vi "test.vi"   [LabVIEW 2015]
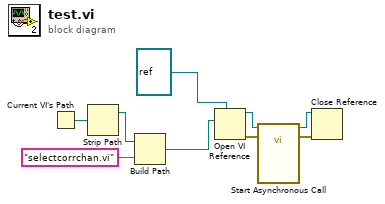
[diagram p0: block diagram]
diagram:
  n1 = Current VI's Path() -> (path=w9:path)
  n2 = Strip Path(path=w9) -> (stripped path=w5:path)  [unwired: 1 out]
  n3 = Build Path(base path=w5, name or relative path="selectcorrchan.vi") -> (appended path=w4:path)
  n4 = Open VI Reference(type specifier VI Refnum (for type only)=refnum<vi> refnum, vi path=w4) -> (vi reference=w2:refnum<vi>, error out=w7:errorcluster)  [unwired: 4 in]
  n5 = call-by-ref "Start Asynchronous Call"(reference=w2, error in=w7) -> (reference out=w1:refnum<vi>, error out=w6:errorcluster)  [unwired: 1 in]
  n6 = Close Reference(reference=w1, error in (no error)=w6) -> ()  [unwired: 1 out]
